vi "ZLIB Enumerate File Contents__ogtk.vi"(8 "error in (no error)":errorcluster, 11 "unzip Refnum":T1) -> (0 "error out":errorcluster, 1 "file infos":T2[](array[typedef]) {"file timestamp" format="%<%H:%M:%S\n%d/%m/%Y>T"; "external fa" format="%.0x"; "internal fa" format="%.0x"; "crc" format="%.0x"}, 2 "file names":string[](array[string]), 3 "unzip Refnum out":T1, 4 "global comment":string)   [LabVIEW 2016]
doc: "Lists all the information contained in the file of an unzip session."
uses:
  <userlib>/_OpenG.lib/lvzip/lvzip.llb/ZLIB File Info__ogtk.ctl
  <userlib>/_OpenG.lib/lvzip/lvzip.llb/ZLIB Unzip Handle__ogtk.ctl
panel:
  # "Please visit http://www.OpenG.org to learn about the\nOpen Source LabVIEW software movement.\n\nNOTICE -- YOU MUST LEAVE THIS NOTICE IN PLACE.  PER THE TERMS OF THE LICENSE BELOW, YOU MAY SUBLICENSE THIS SOFTWARE \nIN ANY WAY THAT DOES NOT CONFLICT WITH THIS LICENSE.\n\n### BSD License (http://www.opensource.org/licenses/bsd-license.php) Begin ###\n \nCopyright (C) 2002-2004 Rolf Kalbermatter rolf.kalbermatter@citeng.com\nCopyright (C) 2002 Jim Kring jim@jimkring.com\n\nAll rights reserved.\n\nRedistribution and use in source and binary forms, with or without modification, are permitted provided that the following conditions are met:\n\n    * Redistributions of source code must retain the above copyright notice, this list of conditions and the following disclaimer.\n    * Redistributions in binary form must reproduce the above copyright notice, this list of conditions and the following disclaimer in the \n       documentation and/or other materials provided with the distribution.\n    * Neither the name of SciWare, James Kring, Inc., nor the names of its contributors may be used to endorse or promote products derived \n       from this software without specific prior written permission.\n\nTHIS SOFTWARE IS PROVIDED BY THE COPYRIGHT HOLDERS AND CONTRIBUTORS \"AS IS\" AND ANY EXPRESS OR IMPLIED WARRANTIES, \nINCLUDING, BUT NOT LIMITED TO, THE IMPLIED WARRANTIES OF MERCHANTABILITY AND FITNESS FOR A PARTICULAR PURPOSE ARE \nDISCLAIMED. IN NO EVENT SHALL THE COPYRIGHT OWNER OR CONTRIBUTORS BE LIABLE FOR ANY DIRECT, INDIRECT, INCIDENTAL,\n SPECIAL, EXEMPLARY, OR CONSEQUENTIAL DAMAGES (INCLUDING, BUT NOT LIMITED TO, PROCUREMENT OF SUBSTITUTE GOODS OR \nSERVICES; LOSS OF USE, DATA, OR PROFITS; OR BUSINESS INTERRUPTION) HOWEVER CAUSED AND ON ANY THEORY OF LIABILITY, \nWHETHER IN CONTRACT, STRICT LIABILITY, OR TORT (INCLUDING NEGLIGENCE OR OTHERWISE) ARISING IN ANY WAY OUT OF THE USE \nOF THIS SOFTWARE, EVEN IF ADVISED OF THE POSSIBILITY OF SUCH DAMAGE.\n\n### BSD License End ###"
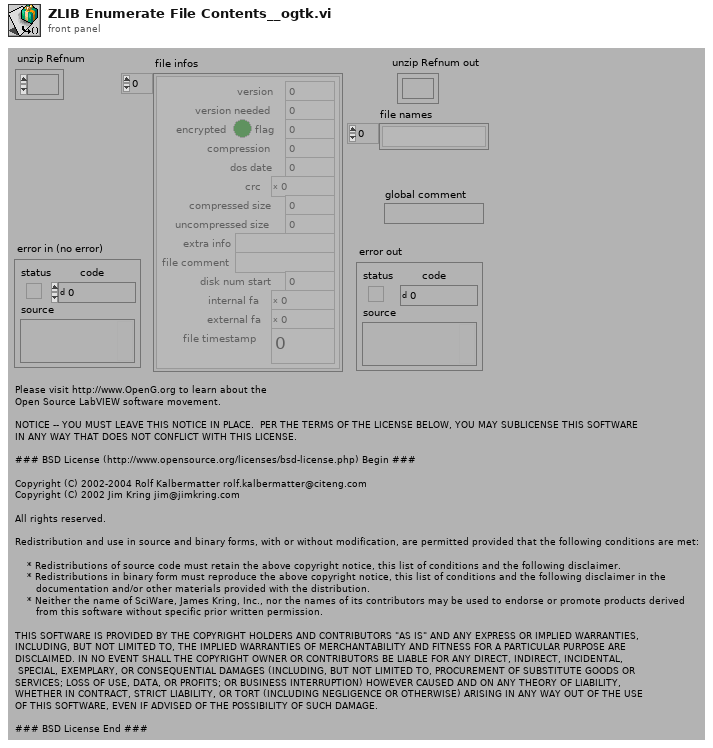
[diagram p1: front panel]
types:
  T1 = typedef "ZLIB Unzip Handle__ogtk.ctl" = refnum<k1>
  T2 = typedef "ZLIB File Info__ogtk.ctl" = cluster{"version":u32, "version needed":u32, "encrypted":bool, "flag":u32, "compression":i32, "dos date":u32, "crc":u32, "compressed size":u32, "uncompressed size":u32, "extra info":string, "file comment":string, "disk num start":u32, "internal fa":u32, "external fa":u32, "file timestamp":u32}
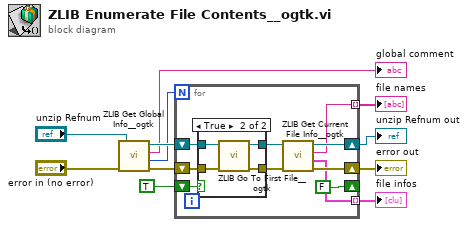
[diagram p0: block diagram]
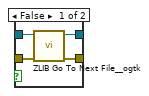
[diagram p2: hidden frame]
diagram:
  n1 = call <userlib>:"ZLIB Get Global Info__ogtk.vi"("error in (no error)"="error in (no error)", "unzip Refnum"="unzip Refnum") -> ("error out"=w11:errorcluster, "nEntry"=w1:u32, "global comment"=→"global comment":string, "unzip Refnum out"=w10:T1)  [unwired: 2 in]
  n2 = for {
    N: w1 -> [_]
    shift-right: [w14] -> w4
    shift-left: w10 -> [w20]
    shift-right: [w15] -> w3
    shift-left: w11 -> [w19]
    shift-right: [FALSE] -> _
    shift-left: TRUE -> [w21]
    tunnel: [w13] -> w8 mode=indexing
    tunnel: [w12] -> w7 mode=indexing
    n3 = case shown="True" w21 {
      tunnel: w20 -> [w24 w29]
      tunnel: w19 -> [w25 w28]
      tunnel: [w23 w27] -> w17
      tunnel: [w22 w26] -> w18
      frame False {
        n4 = call <userlib>:"ZLIB Go To Next File__ogtk.vi"("error in (no error)"=w25, "unzip Refnum"=w24) -> ("error out"=w22:errorcluster, "unzip Refnum out"=w23:T1)  [unwired: 4 in]
      }
      frame True {
        n5 = call <userlib>:"ZLIB Go To First File__ogtk.vi"("error in (no error)"=w28, "unzip Refnum"=w29) -> ("error out"=w26:errorcluster, "unzip Refnum out"=w27:T1)  [unwired: 4 in]
      }
    }
    n6 = call <userlib>:"ZLIB Get Current File Info__ogtk.vi"("error in (no error)"=w18, "unzip Refnum"=w17) -> ("error out"=w15:errorcluster, "file info"=w12:T2, "name"=w13:string, "unzip Refnum out"=w14:T1)  [unwired: 6 in]
  }
  "file names" <- w8
  "file infos" <- w7
  "error out" <- w3
  "unzip Refnum out" <- w4
